vi "PUT (Buffer).vi"(6 "timeout":i32=10000, 7 "output file":path, 8 "error in":errorcluster, 9 "buffer":string, 10 "url":string, 11 "http-method in":refnum<class "REST Client.lvclass">) -> (0 "error out":errorcluster, 2 "response":refnum<class "response.lvclass">, 3 "http-method out":refnum<class "REST Client.lvclass">)   [LabVIEW 2020, in "REST Client.lvlib" / "REST Client.lvclass"]
uses:
  REST Client.lvclass
  response/response.lvclass
  http-client/http-client.lvclass
  REST Client.lvclass/REST Client.ctl
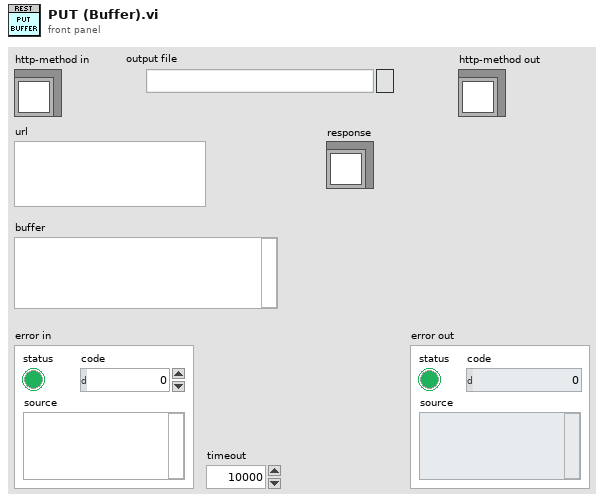
[diagram p1: front panel]
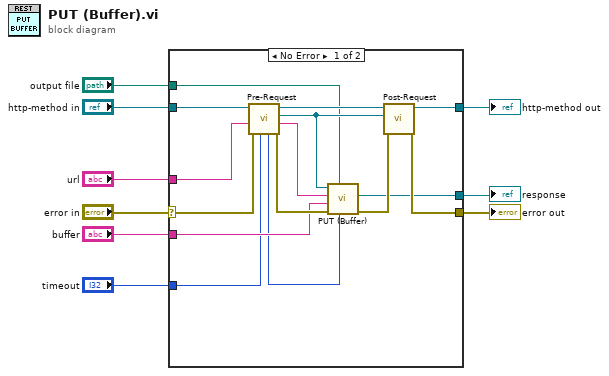
[diagram p0: block diagram]
diagram:
  n1 = case shown="No Error" "error in" {
    selector: "error in" -> [w20 w26]
    tunnel: [w17 w26] -> w8
    tunnel: [w18 w25] -> w7
    tunnel: "http-method in" -> [w19 w25]
    tunnel: "url" -> [w13 _]
    tunnel: "timeout" -> [w11 _]
    tunnel: [w16 _] -> w9
    tunnel: "output file" -> [w15 _]
    tunnel: "buffer" -> [w14 _]
    frame No Error {
      n2 = call "Pre-Request.vi"("timeout"=w11, "error in (no error)"=w20, "url"=w13, "REST Client in"=w19) -> ("error out"=w22:errorcluster, "Resolved URL"=w12:string, "http-client"=w23:refnum<class "http-client.lvclass">, "REST Client out"=w24:refnum<class "REST Client.lvclass">, "Timeout"=w10:i32)  [unwired: 3 in]
      n3 = call-dynamic "PUT (Buffer).vi"("timeout"=w10, "output file"=w15, "error in"=w22, "buffer"=w14, "url"=w12, "http-method in"=w23) -> ("error out"=w21:errorcluster, "response"=w16:refnum<class "response.lvclass">)  [unwired: 3 in, 1 out]
      n4 = call "Post-Request.vi"("error in (no error)"=w21, "http-method in"=w23, "REST Client in"=w24) -> ("error out"=w17:errorcluster, "REST Client out"=w18:refnum<class "REST Client.lvclass">)  [unwired: 7 in]
    }
    frame Error {
    }
  }
  "error out" <- w8
  "http-method out" <- w7
  "response" <- w9
